vi "BAM Generation Queue Messages.vi"(0 "J1939 Cluster":T7, 5 "Connection Refs":T1, 11 "error in":errorcluster) -> (4 "J1939 Cluster Out":T7, 15 "error out":errorcluster)   [LabVIEW 2015, in "J1939 Addon Engine.lvlib"]
uses:
  J1939 Addon Engine.lvlib
  Types/Setup Information Cluster.ctl
  <vilib>/xnet/xnet.llb/XNET Frame CAN.ctl
  <vilib>/xnet/xnet.llb/XNET Frame Type CAN.ctl
  Shared/J1939 Utilities/Types/CAN Outgoing Message Cluster.ctl
  Types/TP List References.ctl
  Types/BAM Buffer Connections List_Ref.ctl
  Types/TP Buffer Connection Cluster.ctl
  Types/Connection Mode Generation Connection Ref.ctl
  Types/Connection Mode Generation Connection Cluster.ctl
  Types/BAM Generation Connections List_Ref.ctl
  Types/BAM Generation Connection Cluster.ctl
  Types/Address Table Reference.ctl
  Types/RQST Lookup Table Reference.ctl
  Types/TP Connections List State.ctl
  BAM Generation Connections List_Actions.vi
  BAM Generation Get Next Message.vi
  BAM Generation Connections List.vi
  Shared/J1939 Utilities/J1939 Utilities.lvlib
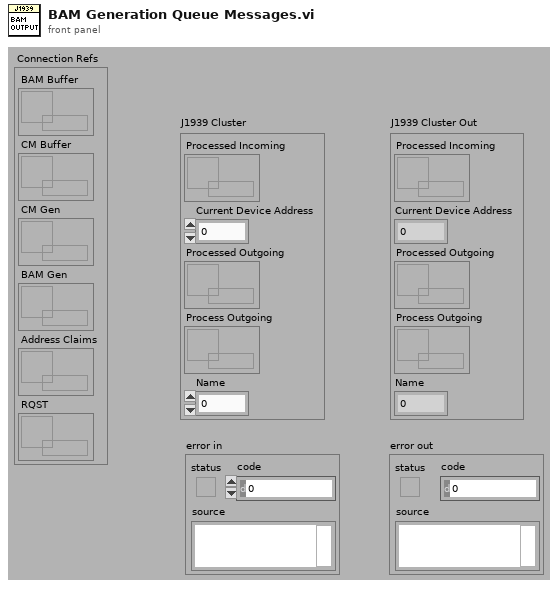
[diagram p1: front panel]
types:
  T1 = typedef "J1939 Addon Engine.lvlib/TP List References.ctl" = cluster{"BAM Buffer":T2, "CM Buffer":T2, "CM Gen":T3, "BAM Gen":T4, "Address Claims":T5, "RQST":T6}
  T2 = typedef "J1939 Addon Engine.lvlib/BAM Buffer Connections List_Ref.ctl" = refnum<data-value>
  T3 = typedef "J1939 Addon Engine.lvlib/Connection Mode Generation Connection Ref.ctl" = refnum<data-value>
  T4 = typedef "J1939 Addon Engine.lvlib/BAM Generation Connections List_Ref.ctl" = refnum<data-value>
  T5 = typedef "J1939 Addon Engine.lvlib/Address Table Reference.ctl" = refnum<data-value>
  T6 = typedef "J1939 Addon Engine.lvlib/RQST Lookup Table Reference.ctl" = refnum<data-value>
  T7 = typedef "J1939 Addon Engine.lvlib/Setup Information Cluster.ctl" = cluster{"Processed Incoming":refnum<queue>, "Current Device Address":u8, "Processed Outgoing":refnum<queue>, "Process Outgoing":refnum<queue>, "Name":u64}
  T8 = typedef "J1939 Addon Engine.lvlib/TP Connections List State.ctl" = enum16{"Add", "Update", "Get", "Remove", "Initialize"}
  T9 = typedef "J1939 Addon Engine.lvlib/BAM Generation Connection Cluster.ctl" = cluster{"Total Packets":u8, "Current Packet to Generate":u8, "Packets":T10[], "Previous Time Stamp":u32, "Total Bytes":u16, "Source Address":u8}
  T10 = typedef "J1939 Addon Shared.lvlib/J1939 Utilities.lvlib/CAN Outgoing Message Cluster.ctl" = cluster{"Identifier":u32, "Data":u8[]}
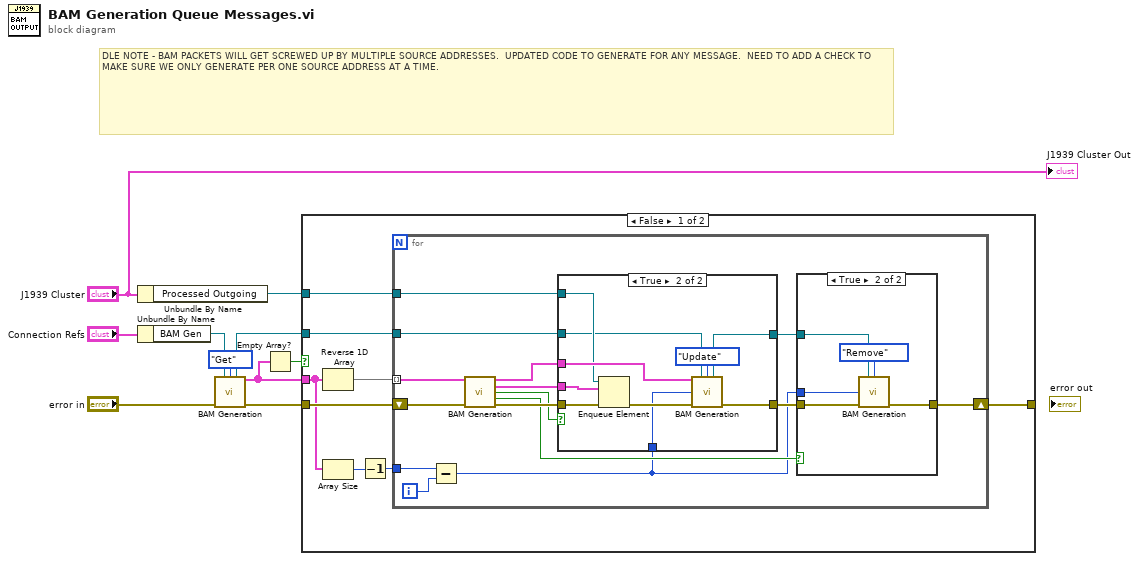
[diagram p0: block diagram]
diagram:
  # "DLE NOTE - BAM PACKETS WILL GET SCREWED UP BY MULTIPLE SOURCE ADDRESSES.  UPDATED CODE TO GENERATE FOR ANY MESSAGE.  NEED TO ADD A CHECK TO MAKE SURE WE ONLY GENERATE PER ONE SOURCE ADDRESS AT A TIME."
  n1 = Unbundle By Name("J1939 Cluster") -> ("Processed Outgoing"=w6:refnum<queue>)
  n2 = Unbundle By Name("Connection Refs") -> ("BAM Gen"=w3:T4)
  n3 = call-poly "BAM Generation.vi"("BAM Gen"=w3, "State"=TP_Connections_List_State."Get", "error in (no error)"="error in") -> ("BAM Gen out"=w2:T4, "Connections"=w1:T9[], "error out"=w8:errorcluster)  [unwired: 2 in, 8 out]
  n4 = Empty Array?(array=w1) -> (empty?=w10:bool)
  n5 = case shown="False" w10 {
    tunnel: w8 -> [w18 w52]
    tunnel: [w17 w52] -> _
    tunnel: w6 -> [w16 _]
    tunnel: w2 -> [w15 _]
    tunnel: w1 -> [w12 _]
    frame False {
      n6 = Reverse 1D Array(array=w12) -> (reversed array=w14:T9[])
      n7 = Array Size(array=w12) -> (size(s)=w13:i32)
      n8 = Decrement(x=w13) -> (x-1=w11:i32)
      n9 = for {
        tunnel: w16 -> [w25]
        tunnel: w15 -> [w24]
        tunnel: w14 -> [w19] mode=indexing
        tunnel: w11 -> [w21]
        shift-right: [w27] -> w17
        shift-left: w18 -> [w33]
        i -> [w22]
        n10 = Subtract(x=w21, y=w22) -> (x-y=w20:i32)
        n11 = call-poly "BAM Generation.vi"("Connecion Cluster"=w19, "error in (no error)"=w33) -> ("Connecion Cluster Out"=w32:T9, "Data to Send"=w30:T10, "Message Available?"=w29:bool, "Message Finished?"=w26:bool, "error out"=w31:errorcluster)  [unwired: 9 out]
        n12 = case shown="True" w29 {
          tunnel: w32 -> [_ w50]
          tunnel: w31 -> [w41 w48]
          tunnel: w30 -> [_ w46]
          tunnel: [w41 w49] -> w28
          tunnel: w25 -> [_ w45]
          tunnel: w24 -> [w40 w44]
          tunnel: [w40 w43] -> w23
          tunnel: w20 -> [_ w42]
          frame False {
          }
          frame True {
            n13 = Enqueue Element(queue=w45, element=w46, error in (no error)=w48) -> (error out=w47:errorcluster)  [unwired: 3 out]
            n14 = call-poly "BAM Generation.vi"("Connection Cluster"=w50, "BAM Gen"=w44, "State"=TP_Connections_List_State."Update", "index"=w42, "error in (no error)"=w47) -> ("BAM Gen out"=w43:T4, "error out"=w49:errorcluster)  [unwired: 9 out]
          }
        }
        n15 = case shown="True" w26 {
          tunnel: w28 -> [w34 w38]
          tunnel: [w34 w37] -> w27
          tunnel: w23 -> [_ w36]
          tunnel: w20 -> [_ w35]
          frame False {
          }
          frame True {
            n16 = call-poly "BAM Generation.vi"("BAM Gen"=w36, "State"=TP_Connections_List_State."Remove", "index"=w35, "error in (no error)"=w38) -> ("error out"=w37:errorcluster)  [unwired: 1 in, 10 out]
          }
        }
      }
    }
    frame True {
    }
  }
  "J1939 Cluster Out" <- "J1939 Cluster"
